vi "AttackerAvoidArea.vi"(9 "AttackerAvoidArea":bool=TRUE, 10 "obstacle enemy radius":dbl, 11 "array in":dbl[][](array[numeric])) -> (3 "array out":dbl[][](array[numeric]))   [LabVIEW 2023]
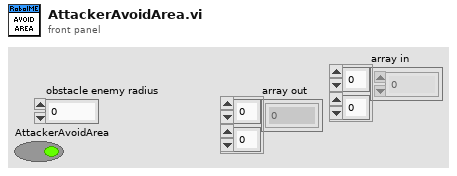
[diagram p1: front panel]
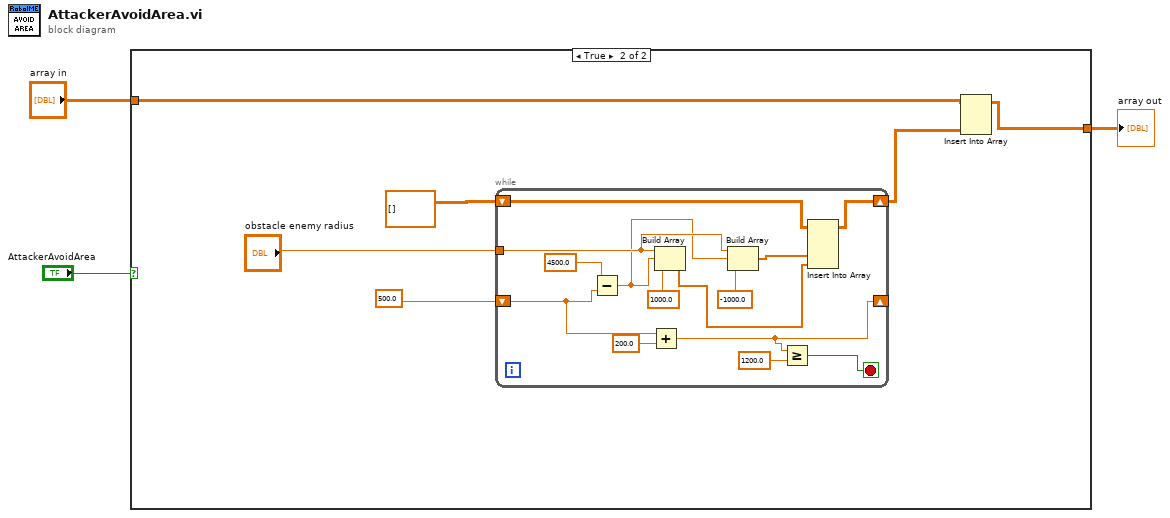
[diagram p0: block diagram]
diagram:
  n1 = case shown="True" "AttackerAvoidArea" {
    tunnel: "array in" -> [w4 w7]
    tunnel: [w4 w5] -> w2
    frame False {
    }
    frame True {
      n2 = while {
        tunnel: "obstacle enemy radius" -> [w16]
        shift-right: [w20] -> _
        shift-left: 500.0 -> [w22]
        shift-right: [w11] -> w6
        shift-left: dbl[][] [] ("array") -> [w14]
        stop <- w18 stop-if-true
        n3 = Subtract(x=4500.0 ("element"), y=w22) -> (x-y=w15:dbl)
        n4 = Add(x=w22, y=200.0) -> (x+y=w20:dbl)
        n5 = Build Array(w16, w15, 1000.0 ("element")) -> (w12:dbl[])
        n6 = Build Array(w16, w15, -1000.0 ("element")) -> (w13:dbl[])
        n7 = Greater Or Equal?(x=w20, y=1200.0) -> (x >= y?=w18:bool)
        n8 = Insert Into Array(array=w14, new element #1=w13, new element #2=w12) -> (w11:dbl[][])  [unwired: 2 in]
      }
      n9 = Insert Into Array(array=w7, new element=w6) -> (w5:dbl[][])  [unwired: 2 in]
    }
  }
  "array out" <- w2
